vi "Merge Errors with Paths.vi"(8 "Errors":errorcluster[](array[cluster]), 10 "Relative File Paths In":string[](array[string])) -> (0 "error out":errorcluster, 2 "Relative File Paths Out":string[](array[string]))   [LabVIEW 2017, in "XTree.xctl"]
doc: "Combines errors from the Add File to Tree SubVI so that if an error is returned from opening a file, the file name will be appended to the error source. In addition, that file is removed from the list so access will not be attempted again."
uses:
  <vilib>/addons/_NIFileIO/XTree/XTree.xctl
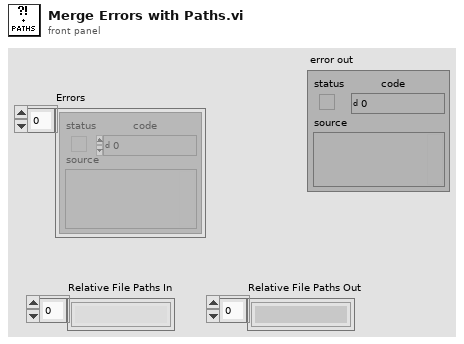
[diagram p1: front panel]
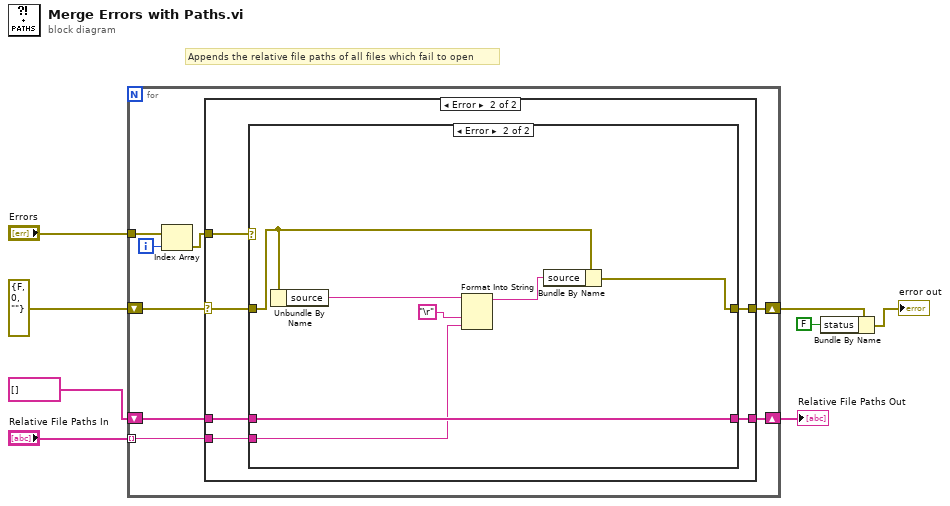
[diagram p0: block diagram]
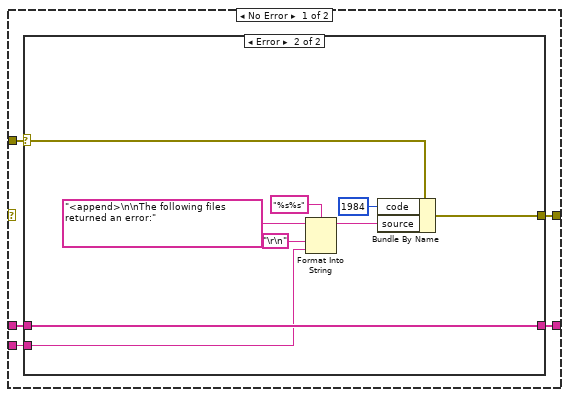
[diagram p2: hidden frame]
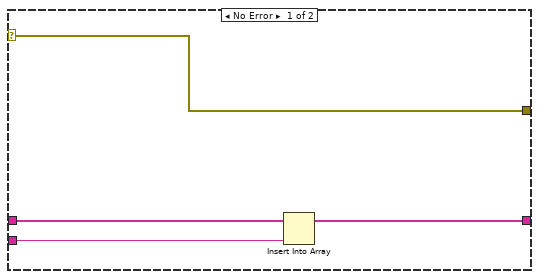
[diagram p3: hidden frame]
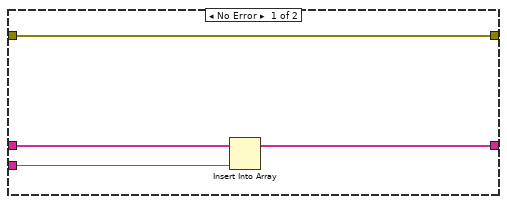
[diagram p4: hidden frame]
diagram:
  # "Appends the relative file paths of all files which fail to open"
  n1 = for {
    shift-right: [w15] -> w3
    shift-left: errorcluster {"status"=FALSE, "code"=0, "source"=""} ("error constant") -> [w16]
    tunnel: "Errors" -> [w12]
    tunnel: "Relative File Paths In" -> [w9] mode=indexing
    shift-right: [w13] -> w4
    shift-left: string[] [] -> [w14]
    i -> [w11]
    n2 = Index Array(array=w12, index=w11) -> (element=w10:errorcluster)
    n3 = case shown="Error" w16 {
      selector: w16 -> [_ w39]
      tunnel: w10 -> [w21 w40]
      tunnel: [w20 w38] -> w15
      tunnel: w14 -> [w19 w37]
      tunnel: [w18 w36] -> w13
      tunnel: w9 -> [w17 w35]
      frame No Error {
        n4 = case shown="Error" w21 {
          selector: w21 -> [w25 w34]
          tunnel: [w25 w33] -> w20
          tunnel: w19 -> [w23 w28]
          tunnel: [w22 w28] -> w18
          tunnel: w17 -> [w24 w27]
          frame No Error {
            n5 = Insert Into Array(array=w23, new element=w24) -> (w22:string[])  [unwired: 1 in]
          }
          frame Error {
            n6 = Format Into String(format string="%s%s", initial string="<append>\n\nThe following files returned an error:" ("source"), "\r\n", w27) -> (resulting string=w31:string)  [unwired: 1 in, 1 out]
            n7 = Bundle By Name(cluster=w34, "code"=1984, "source"=w31) -> (w33:errorcluster)
          }
        }
      }
      frame Error {
        n8 = case shown="Error" w40 {
          tunnel: w39 -> [w44 w49]
          tunnel: [w44 w50] -> w38
          tunnel: w37 -> [w43 w46]
          tunnel: [w42 w46] -> w36
          tunnel: w35 -> [w41 w45]
          frame No Error {
            n9 = Insert Into Array(array=w43, new element=w41) -> (w42:string[])  [unwired: 1 in]
          }
          frame Error {
            n10 = Unbundle By Name(w49) -> ("source"=w48:string)
            n11 = Format Into String(initial string=w48, "\r", w45) -> (resulting string=w51:string)  [unwired: 2 in, 1 out]
            n12 = Bundle By Name(cluster=w49, "source"=w51) -> (w50:errorcluster)
          }
        }
      }
    }
  }
  "Relative File Paths Out" <- w4
  n13 = Bundle By Name(cluster=w3, "status"=FALSE) -> (→"error out":errorcluster)
